vi "Read configuration.vi"(8 "error in":errorcluster, 11 "sbRIO-9651 in":refnum<class "sbRIO-9651.lvclass">) -> (0 "error out":errorcluster, 2 "configuration":refnum<class "NISE_CEF_serializable configuration.lvclass">, 3 "sbRIO-9651 out":refnum<class "sbRIO-9651.lvclass">)   [LabVIEW 2014, in "sbRIO-9651.lvclass"]
uses:
  sbRIO-9651.lvclass
  <vilib>/NI/Configuration Framework/serializable configuration/NISE_CEF_serializable configuration.lvclass
  sbRIO-9651.lvclass/sbRIO-9651.ctl
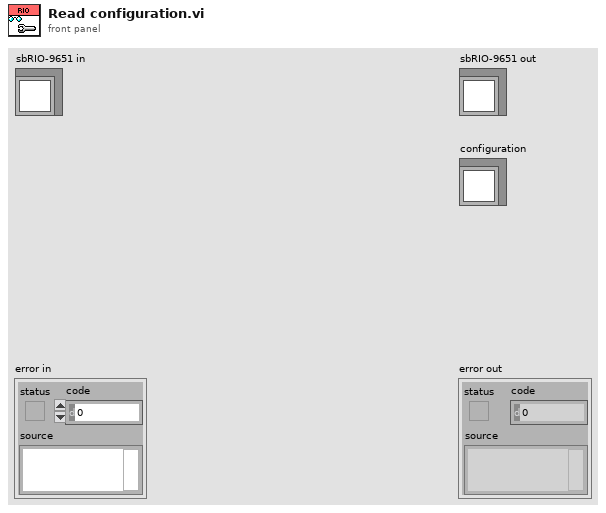
[diagram p1: front panel]
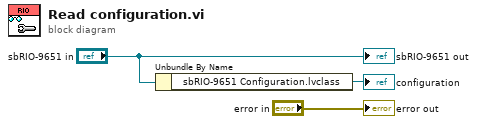
[diagram p0: block diagram]
diagram:
  n1 = Unbundle By Name("sbRIO-9651 in") -> ("sbRIO-9651 Configuration.lvclass"=→"configuration":refnum<class "sbRIO-9651 Configuration.lvclass">)
  "error out" <- "error in"
  "sbRIO-9651 out" <- "sbRIO-9651 in"
